vi "Configure.vi"(8 "error in (no error)":errorcluster, 9 "Default Path":path, 10 "Interactive?":bool, 11 "XML Report In":refnum<class "Coverage Report.lvclass">) -> (0 "error out":errorcluster, 3 "XML Report Out":refnum<class "Coverage Report.lvclass">)   [LabVIEW 2020, in "Coverage Report.lvclass"]
uses:
  Coverage Report.lvclass
  Coverage Report.lvclass/Coverage Report.ctl
  User Interface/Configuration Manager/Configuration Manager.lvclass
  User Interface/Support/Paths.lvlib
panel:
  in  "Cancel":bool
  in  "Commit":bool
  in  "Open New Reports":bool
  in  "Report Path":path
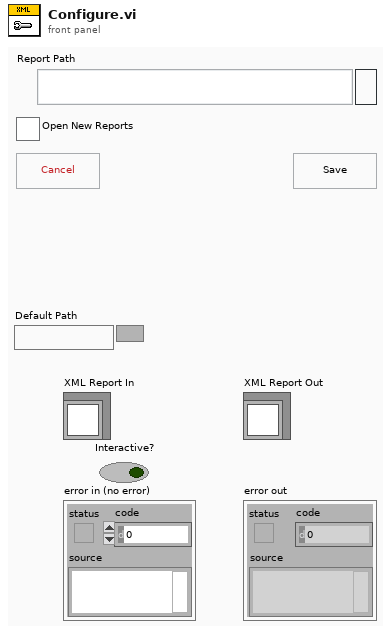
[diagram p1: front panel]
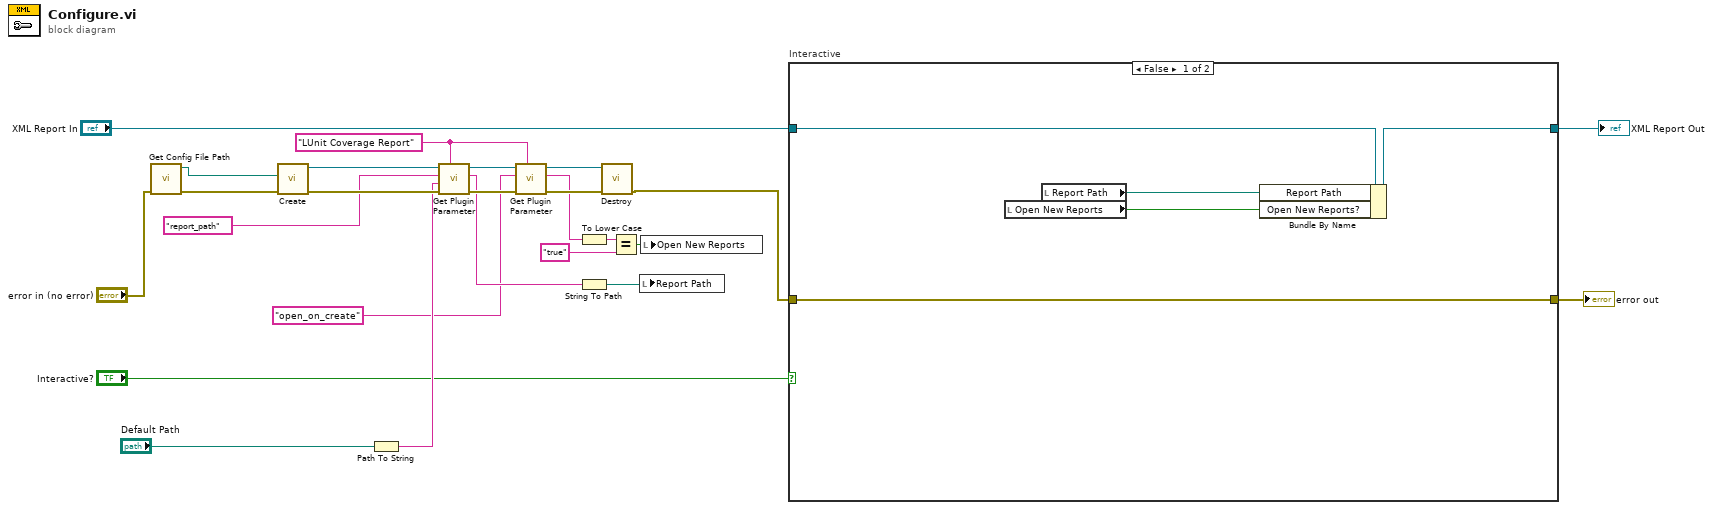
[diagram p0: block diagram]
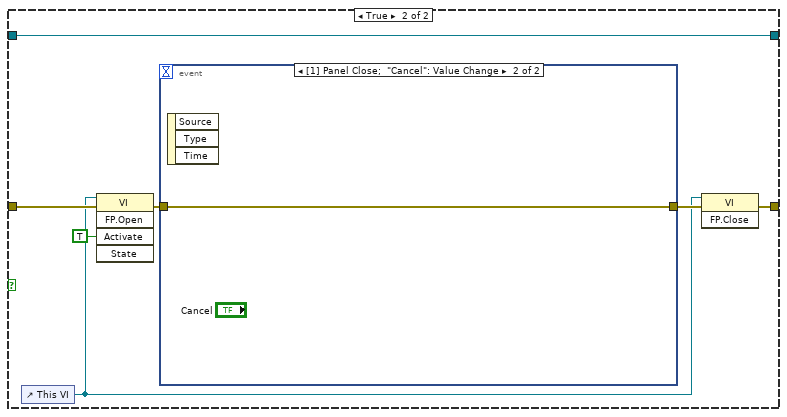
[diagram p2: hidden frame]
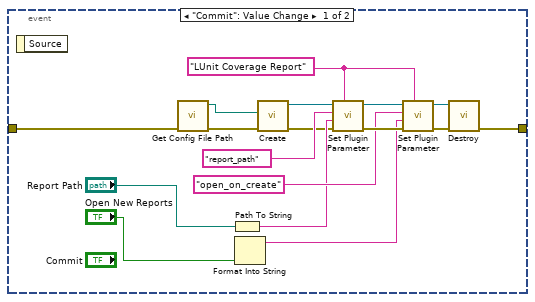
[diagram p3: hidden frame]
diagram:
  w8 = "LUnit Coverage Report"
  n1 = call "Get Config File Path.vi"("error in (no error)"="error in (no error)") -> ("error out"=w24:errorcluster, "Config Directory"=w23:path)  [unwired: 9 in]
  n2 = call "Create.vi"("error in (no error)"=w24, "configuration file path"=w23) -> ("error out"=w21:errorcluster, "Configuration Manager out"=w25:refnum<class "Configuration Manager.lvclass">)  [unwired: 8 in]
  n3 = Path To String(path="Default Path") -> (string=w19:string)
  n4 = call "Get Plugin Parameter.vi"("Plugin"=w8, "error in (no error)"=w21, "Default Value"=w19, "Name"="report_path", "Configuration Manager in"=w25) -> ("error out"=w22:errorcluster, "Value"=w17:string, "Configuration Manager out"=w15:refnum<class "Configuration Manager.lvclass">)  [unwired: 4 in]
  n5 = call "Get Plugin Parameter.vi"("Plugin"=w8, "error in (no error)"=w22, "Name"="open_on_create", "Configuration Manager in"=w15) -> ("error out"=w16:errorcluster, "Value"=w12:string, "Configuration Manager out"=w14:refnum<class "Configuration Manager.lvclass">)  [unwired: 5 in]
  n6 = To Lower Case(string=w12) -> (all lower case string=w11:string)
  n7 = String To Path(string=w17) -> (path=w18:path)
  n8 = call "Destroy.vi"("error in (no error)"=w16, "Configuration Manager In"=w14) -> ("error out"=w6:errorcluster)  [unwired: 9 in]
  n9 = Equal?(x=w11, y="true") -> (x = y?=w9:bool)
  n10 = local write "Report Path"(w18) -> ()
  n11 = local write "Open New Reports"(w9) -> ()
  n12 = case "Interactive" shown="False" "Interactive?" {
    tunnel: w6 -> [w30 w35]
    tunnel: [w30 w33] -> w5
    tunnel: "XML Report In" -> [w29 w31]
    tunnel: [w28 w31] -> w2
    frame False {
      n13 = local read "Open New Reports"() -> (w26:bool)
      n14 = local read "Report Path"() -> (w27:path)
      n15 = Bundle By Name(cluster=w29, "Report Path"=w27, "Open New Reports?"=w26) -> (w28:refnum<class "Coverage Report.lvclass">)
    }
    frame True {
      n16 = control-ref of="This VI"() -> (w32:refnum<vi>)
      n17 = invoke class="VI" method="FP.Open"(reference=w32, error in=w35, "Activate"=TRUE ("Activate?")) -> (error out=w36:errorcluster)  [unwired: 2 in, 4 out]
      n18 = event shown="[1] Panel Close;  \"Cancel\": Value Change" {
        selector: _ -> [_ _]
        dyn-events: _ -> [_ _]
        timeout: _ -> [_ _]
        tunnel: w36 -> [w54 w55]
        tunnel: [w53 w55] -> w34
        event "Commit": Value Change {
          w52 = "LUnit Coverage Report"
          n19 = event-data() -> ()  [unwired: 1 in, 1 out]
          n20 = call "Get Config File Path.vi"("error in (no error)"=w54) -> ("error out"=w45:errorcluster, "Config Directory"=w44:path)  [unwired: 9 in]
          n21 = Path To String(path="Report Path") -> (string=w47:string)
          n22 = Format Into String("Open New Reports") -> (resulting string=w46:string)  [unwired: 3 in, 1 out]
          n23 = call "Create.vi"("error in (no error)"=w45, "configuration file path"=w44) -> ("error out"=w42:errorcluster, "Configuration Manager out"=w43:refnum<class "Configuration Manager.lvclass">)  [unwired: 8 in]
          n24 = call "Set Plugin Parameter.vi"("Plugin"=w52, "error in (no error)"=w42, "Value"=w47, "Name"="report_path", "Configuration Manager in"=w43) -> ("error out"=w50:errorcluster, "Configuration Manager out"=w51:refnum<class "Configuration Manager.lvclass">)  [unwired: 5 in]
          n25 = call "Set Plugin Parameter.vi"("Plugin"=w52, "error in (no error)"=w50, "Value"=w46, "Name"="open_on_create", "Configuration Manager in"=w51) -> ("error out"=w40:errorcluster, "Configuration Manager out"=w41:refnum<class "Configuration Manager.lvclass">)  [unwired: 5 in]
          n26 = call "Destroy.vi"("error in (no error)"=w40, "Configuration Manager In"=w41) -> ("error out"=w53:errorcluster)  [unwired: 9 in]
        }
        event Panel Close; "Cancel": Value Change {
          n27 = event-data() -> ()  [unwired: 1 in, 3 out]
        }
      }
      n28 = invoke class="VI" method="FP.Close"(reference=w32, error in=w34) -> (error out=w33:errorcluster)  [unwired: 1 in, 2 out]
    }
  }
  "error out" <- w5
  "XML Report Out" <- w2
